vi "Delete Mapping.vi"(8 "error in (no error)":errorcluster, 10 "Row Name":string, 11 "references":T1) -> (0 "error out":errorcluster, 3 "references out":T1)   [LabVIEW 2013, in "Scaling editor node.lvclass"]
uses:
  Scaling editor node.lvclass
  <vilib>/NI/DCAF Table API/Table Manager/object ref.ctl
  <vilib>/NI/DCAF/Tag Editor Core/Configuration Editor/Classes/Engine Parent/Engine Parent Editor Node.lvclass
  <vilib>/NI/DCAF/Tag Editor Core/Configuration Editor/Classes/Module editor node/module editor node.lvclass
  module/configuration/Scaling configuration.lvclass
  <vilib>/NI/DCAF Table API/Table Manager/Table Manager.lvclass
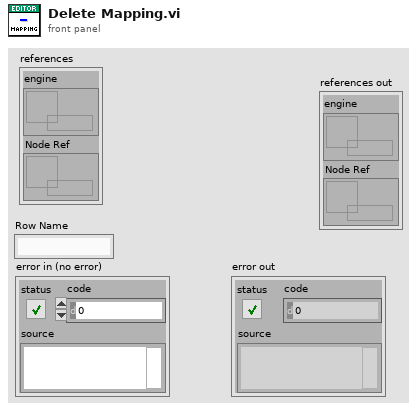
[diagram p1: front panel]
types:
  T1 = typedef "Table Manager.lvlib/Table Manager.lvclass/object ref.ctl" = cluster{"engine":refnum<data-value>, "Node Ref":refnum<data-value>}
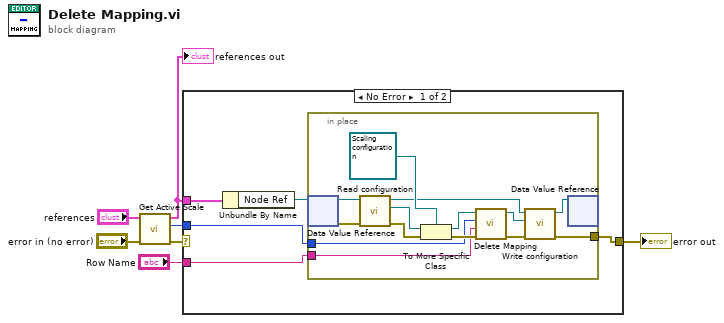
[diagram p0: block diagram]
diagram:
  n1 = call "Get Active Scale.vi"("error in (no error)"="error in (no error)", "references"="references") -> ("error out"=w3:errorcluster, "Index"=w2:i32, "references out"=w4:T1)  [unwired: 6 in]
  "references out" <- w4
  n2 = case shown="No Error" w3 {
    selector: w3 -> [_ w27]
    tunnel: [w12 w27] -> w7
    tunnel: w4 -> [w10 _]
    tunnel: w2 -> [w9 _]
    tunnel: "Row Name" -> [w8 _]
    frame No Error {
      n3 = Unbundle By Name(w10) -> ("Node Ref"=w11:refnum<data-value>)
      n4 = in-place {
        in-place-border: [w19] -> w12
        in-place-border: w9 -> [w14]
        in-place-border: w8 -> [w13]
        n5 = in-place-dvr #1(w11) -> (w17:refnum<class "module editor node.lvclass">, w26:errorcluster)
        n6 = call-dynamic "Read configuration.vi"("error in"=w26, "NISE_CEF_serializable node in"=w17) -> ("error out"=w23:errorcluster, "configuration"=w25:refnum<class "NISE_CEF_serializable configuration.lvclass">, "NISE_CEF_serializable node out"=w16:refnum<class "module editor node.lvclass">)  [unwired: 7 in]
        n7 = To More Specific Class(target class=refnum<class "Scaling configuration.lvclass"> refnum ("Scaling configuration"), reference=w25, error in=w23) -> (specific class reference=w22:refnum<class "Scaling configuration.lvclass">, error out=w21:errorcluster)
        n8 = call "Delete Mapping.vi"("error in (no error)"=w21, "row name"=w13, "scale index"=w14, "Scaling configuration in"=w22) -> ("error out"=w18:errorcluster, "Scaling configuration out"=w20:refnum<class "Scaling configuration.lvclass">)  [unwired: 6 in]
        n9 = call-dynamic "Write configuration.vi"("error in"=w18, "configuration"=w20, "NISE_CEF_serializable node in"=w16) -> ("error out"=w19:errorcluster, "NISE_CEF_serializable node out"=w15:refnum<class "module editor node.lvclass">)  [unwired: 7 in]
        n10 = in-place-dvr #1(w15) -> ()  [unwired: 2 out]
      }
    }
    frame Error {
    }
  }
  "error out" <- w7
